vi "Trim_Whitespace_re_entrant.vi"(1 "location (both)":u16(ring) items=["both", "start of string", "end of string"], 3 "string":string) -> (0 "trimmed string":string)   [LabVIEW 2015]
doc: "Removes all ASCII white space (space, tabs, carriage returns, and linefeeds) from the beginning, end, or both ends of <b>string</b>. The Trim Whitespace VI does not remove double byte characters.\n\nAdditionaly, is set to Shared clone reentrant execution."
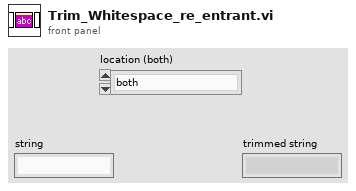
[diagram p1: front panel]
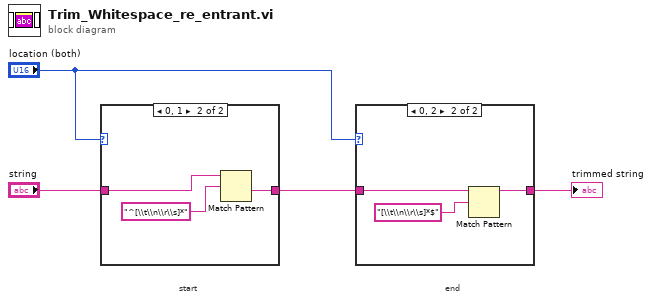
[diagram p0: block diagram]
diagram:
  # "end"
  # "start"
  n1 = case shown="0, 1" "location (both)" {
    tunnel: "string" -> [w5 w6]
    tunnel: [w5 w8] -> w2
    frame Default {
    }
    frame 0, 1 {
      n2 = Match Pattern(string=w6, regular expression="^[\\t\\n\\r\\s]*") -> (after substring=w8:string)  [unwired: 1 in, 3 out]
    }
  }
  n3 = case shown="0, 2" "location (both)" {
    tunnel: w2 -> [w9 w10]
    tunnel: [w9 w11] -> w1
    frame Default {
    }
    frame 0, 2 {
      n4 = Match Pattern(string=w10, regular expression="[\\t\\n\\r\\s]*$") -> (before substring=w11:string)  [unwired: 1 in, 3 out]
    }
  }
  "trimmed string" <- w1
